vi "Init Runtime.vi"(8 "error in (no error)":errorcluster, 10 "data allocations":T1, 11 "String Compare Config in":refnum<class "String Compare Config.lvclass">) -> (0 "error out":errorcluster, 2 "Skip":bool, 3 "String Compare Config out":refnum<class "String Compare Config.lvclass">)   [LabVIEW 2015, in "String Compare Config.lvclass"]
uses:
  String Compare Config.lvclass
  <vilib>/NI/Tag Bus Module Framework/channel/data tables.ctl
  <vilib>/NI/Tag Bus/dictionary/data dictionary.lvclass
  <vilib>/NI/Tag Bus/dictionary table pair.ctl
  <vilib>/NI/Tag Bus/table/data table.ctl
  Runtime/String Compare.lvclass
  String Compare Config.lvclass/String Compare Config.ctl
  <vilib>/NI/Tag Bus/tag/tag descriptor.lvclass/tag descriptor.ctl
  Runtime/String Compare.lvclass/String Compare.ctl
  Read Test Value Channel.vi
  Read Result Channel.vi
  Read Mode.vi
  Read Limit_Regex.vi
  Read Ignore Case.vi
  Read Multiline.vi
  Read offset.vi
  Runtime/Write Test Value Channel Index.vi
  Runtime/Write Result Channel Index.vi
  Runtime/Write Mode.vi
  Runtime/Write Limit_Regex.vi
  Runtime/Write Ignore Case.vi
  Runtime/Write Multiline.vi
  Runtime/Write Offset.vi
  <vilib>/NI/Tag Bus/tag/read tag name.vi
  <vilib>/NI/Tag Bus/tag/read data type.vi
  <vilib>/NI/Tag Bus/dictionary/locate tag.vi
  <vilib>/NI/Tag Bus Module Framework/channel/TBM channel.lvclass
  <vilib>/NI/Tag Bus/table/data table.lvlib
  <vilib>/NI/Tag Bus/tag bus.lvlib
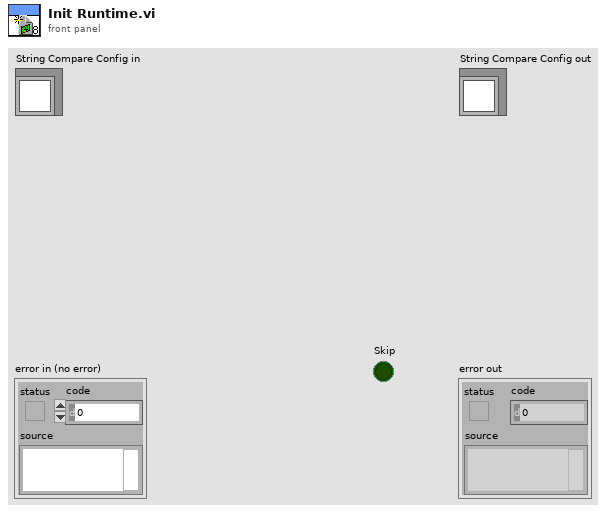
[diagram p1: front panel]
types:
  T1 = typedef "TBM channel.lvclass/data tables.ctl" = cluster{"input data":T2, "processing parameter":T2, "processing result":T2, "output data":T2}
  T2 = typedef "tag bus.lvlib/dictionary table pair.ctl" = cluster{"data dictionary":refnum<class "data dictionary.lvclass">, "data table":T3}
  T3 = typedef "tag bus.lvlib/data table.lvlib/data table.ctl" = cluster{"Double":dbl[], "Single":sgl[], "I64":i64[], "I32":i32[], "I16":i16[], "I8":i8[], "U64":u64[], "U32":u32[], "U16":u16[], "U8":u8[], "Boolean":bool[], "String":string[], "Array of Double":cluster{"DBL Array":dbl[]}[], "Array of Single":cluster{"SGL Array":sgl[]}[], "Array of I64":cluster{"I64 Array":i64[]}[], "Array of I32":cluster{"I32 Array":i32[]}[], "Array of I16":cluster{"I16 Array":i16[]}[], "Array of I8":cluster{"I8 Array":i8[]}[], "Array of U64":cluster{"U64 Array":u64[]}[], "Array of U32":cluster{"U32 Array":u32[]}[], "Array of U16":cluster{"U16 Array":u16[]}[], "Array of U8":cluster{"U8 Array":u8[]}[], "Array of Boolean":cluster{"Boolean Array":bool[]}[], "Array of String":cluster{"String Array":string[]}[]}
  T4 = typedef "Mode.ctl" = enum16{"Compare Strings", "Match Regex"}
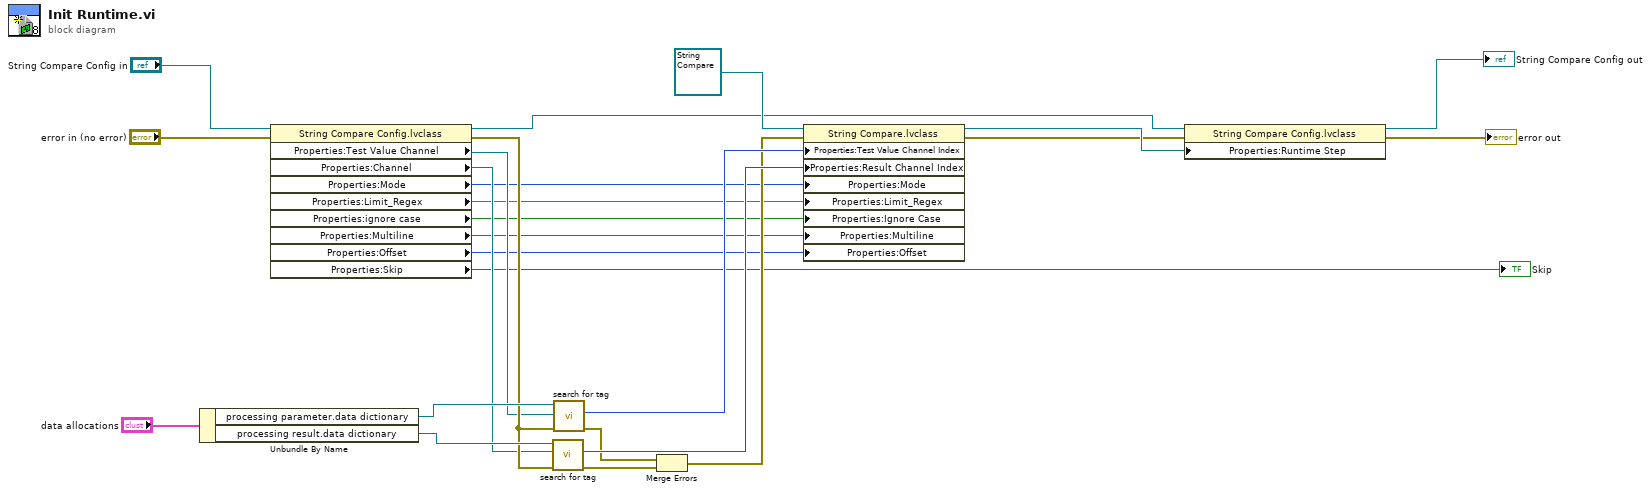
[diagram p0: block diagram]
diagram:
  n1 = Unbundle By Name("data allocations") -> ("processing parameter.data dictionary"=w23:refnum<class "data dictionary.lvclass">, "processing result.data dictionary"=w22:refnum<class "data dictionary.lvclass">)
  n2 = property class="String Compare Config.lvclass"(reference="String Compare Config in", error in="error in (no error)") -> (reference out=w5:refnum<class "String Compare Config.lvclass">, error out=w19:errorcluster, "Properties:Test Value Channel"=w18:refnum<class "TBM channel.lvclass">, "Properties:Channel"=w17:refnum<class "TBM channel.lvclass">, "Properties:Mode"=w11:T4, "Properties:Limit_Regex"=w10:string, "Properties:ignore case"=w9:bool, "Properties:Multiline"=w8:bool, "Properties:Offset"=w7:i32, "Properties:Skip"=→"Skip":bool)
  n3 = call <vilib>:"search for tag.vi"("error in"=w19, "system tag"=w17, "data dictionary in"=w22) -> ("error out"=w14:errorcluster, "index"=w15:i32)  [unwired: 6 in, 1 out]
  n4 = call <vilib>:"search for tag.vi"("error in"=w19, "system tag"=w18, "data dictionary in"=w23) -> ("error out"=w13:errorcluster, "index"=w16:i32)  [unwired: 6 in, 1 out]
  n5 = Merge Errors(w13, w14) -> (w12:errorcluster)
  n6 = property class="String Compare.lvclass"(reference=refnum<class "String Compare.lvclass"> refnum ("String Compare.lvclass"), error in=w12, "Properties:Test Value Channel Index"=w16, "Properties:Result Channel Index"=w15, "Properties:Mode"=w11, "Properties:Limit_Regex"=w10, "Properties:Ignore Case"=w9, "Properties:Multiline"=w8, "Properties:Offset"=w7) -> (reference out=w4:refnum<class "String Compare.lvclass">, error out=w3:errorcluster)
  n7 = property class="String Compare Config.lvclass"(reference=w5, error in=w3, "Properties:Runtime Step"=w4) -> (reference out=→"String Compare Config out":refnum<class "String Compare Config.lvclass">, error out=→"error out":errorcluster)
